vi "Utils - ConvertBitmaptoByteArray.vi"(8 "error in (no error)":errorcluster, 11 "Bitmap image":refnum<k24>) -> (0 "error out":errorcluster, 3 "1DImageData":u8[](array[numeric]))   [LabVIEW 2013]
doc: "Convert .Net Bitmap Image to 1D u8 image data. xiAPI Does not use this method. The continuously lock and unlock procedure takes long. Please use Utils - Convert1DImageToLVImage.vi"
uses:
  System.Drawing
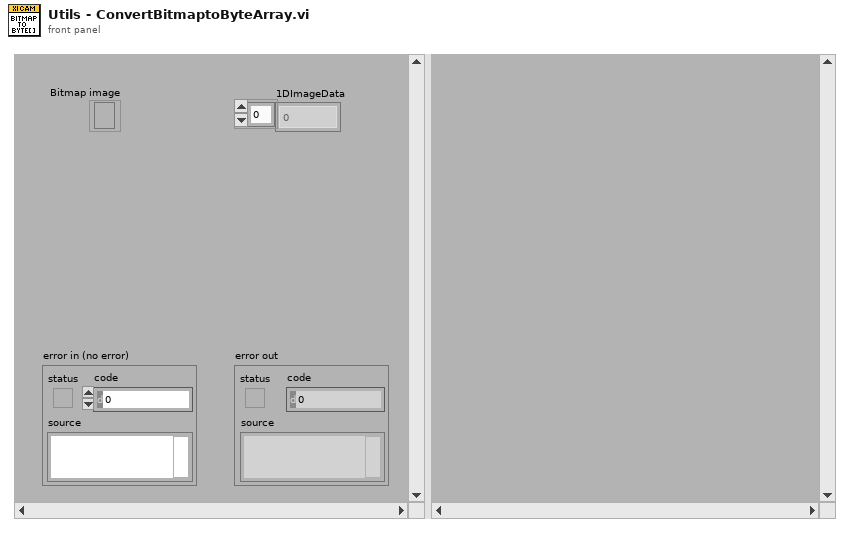
[diagram p1: front panel]
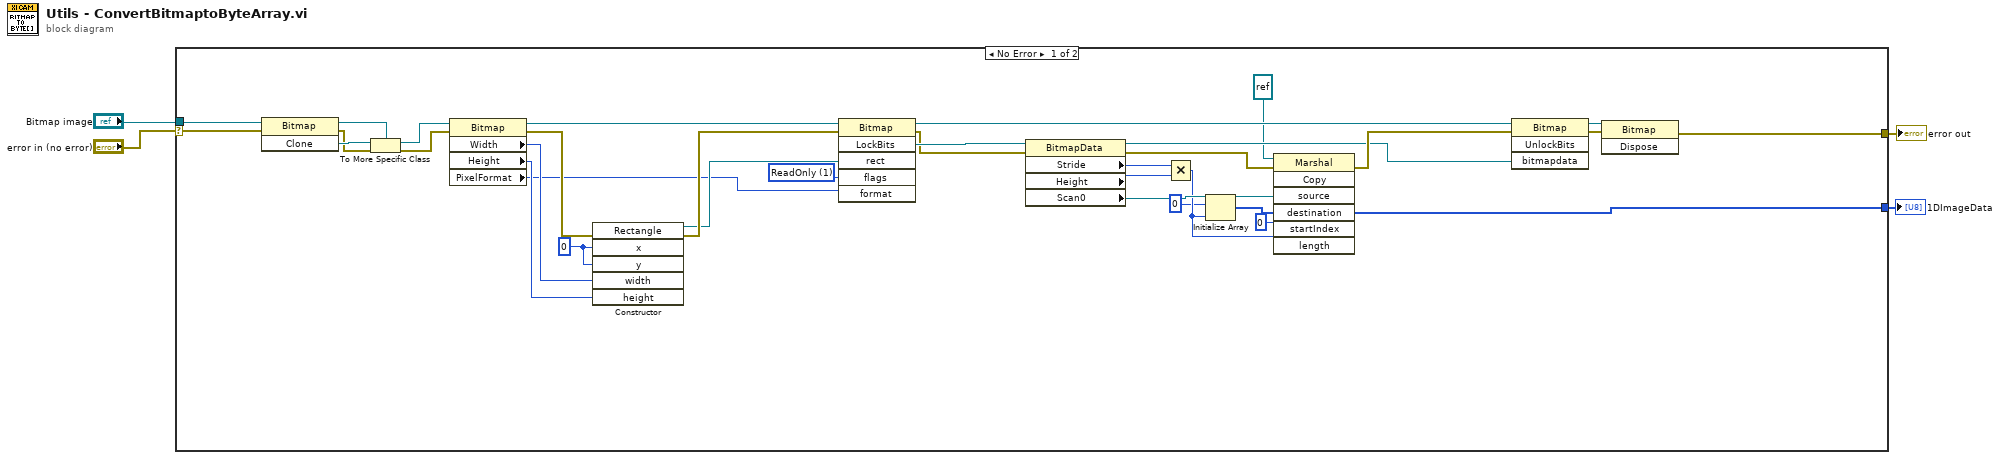
[diagram p0: block diagram]
diagram:
  n1 = case shown="No Error" "error in (no error)" {
    selector: "error in (no error)" -> [w34 w39]
    tunnel: "Bitmap image" -> [w35 _]
    tunnel: [w33 w39] -> w2
    tunnel: [w32 _] -> w1
    frame No Error {
      w11 = 1 items=["ReadOnly"=1, "WriteOnly"=2, "ReadWrite"=3, "UserInputBuffer"=4] ("flags")
      w10 = 0 ("x")
      n2 = invoke class="Bitmap" method="Clone"(reference=w35, error in=w34) -> (reference out=w19:refnum<k24>, error out=w18:errorcluster, "Clone"=w20:refnum<k24>)  [unwired: 1 in]
      n3 = To More Specific Class(target class=w19, reference=w20, error in=w18) -> (specific class reference=w16:refnum<k24>, error out=w17:errorcluster)
      n4 = property class="Bitmap"(reference=w16, error in=w17) -> (reference out=w14:refnum<k24>, error out=w15:errorcluster, "Width"=w9:i32, "Height"=w8:i32, "PixelFormat"=w7:i32)
      n5 = constructor class="Rectangle"(error in=w15, "x"=w10, "y"=w10, "width"=w9, "height"=w8) -> (reference out=w12:refnum<k24>, error out=w13:errorcluster)  [unwired: 2 in, 5 out]
      n6 = invoke class="Bitmap" method="LockBits"(reference=w14, error in=w13, "rect"=w12, "flags"=w11, "format"=w7) -> (reference out=w37:refnum<k24>, error out=w30:errorcluster, "LockBits"=w31:refnum<k24>)  [unwired: 1 in, 3 out]
      n7 = property class="BitmapData"(reference=w31, error in=w30) -> (reference out=w36:refnum<k24>, error out=w25:errorcluster, "Stride"=w21:i32, "Height"=w22:i32, "Scan0"=w29:refnum<k24>)
      n8 = Multiply(x=w21, y=w22) -> (x*y=w24:i32)
      n9 = Initialize Array(u8 0 ("dimension size"), w24) -> (w27:u8[])
      n10 = invoke class="Marshal" method="Copy"(reference=refnum<k24> refnum ("reference out"), error in=w25, "source"=w29, "destination"=w27, "startIndex"=0, "length"=w24) -> (error out=w38:errorcluster, "destination"=w32:u8[])  [unwired: 1 in, 5 out]
      n11 = invoke class="Bitmap" method="UnlockBits"(reference=w37, error in=w38, "bitmapdata"=w36) -> (reference out=w5:refnum<k24>, error out=w6:errorcluster)  [unwired: 1 in, 2 out]
      n12 = invoke class="Bitmap" method="Dispose"(reference=w5, error in=w6) -> (error out=w33:errorcluster)  [unwired: 1 in, 2 out]
    }
    frame Error {
    }
  }
  "error out" <- w2
  "1DImageData" <- w1
